vi "Parse Headers.vi"(8 "error in":errorcluster, 11 "Header-Body Data in":T1) -> (0 "error out":errorcluster, 2 "HTTP Status":T2, 3 "Header-Body Data out":T1)   [LabVIEW 2020, in "InfluxDB v2 Client.lvlib"]
doc: "Parses headers into the components:\n1) Code\n2) Status (Headers)"
uses:
  InfluxDB v2 Client.lvlib
  HTTP Status.ctl
  Header-Body Data.ctl
  <vilib>/regexp/Match Regular Expression.xnode
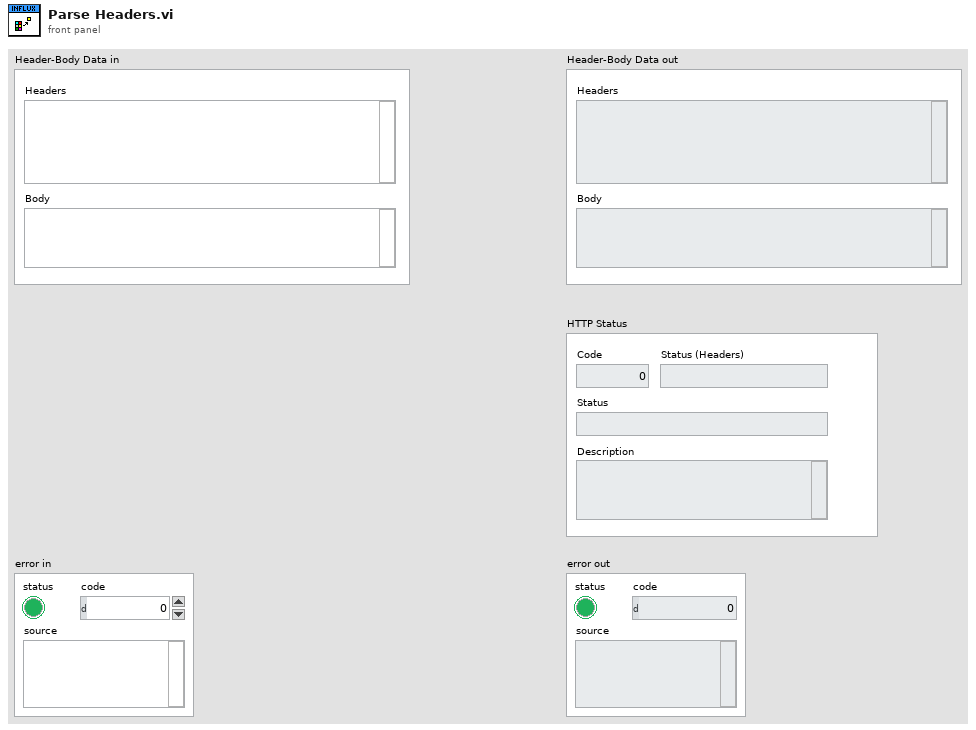
[diagram p1: front panel]
types:
  T1 = typedef "InfluxDB v2 Client.lvlib/Header-Body Data.ctl" = cluster{"Headers":string, "Body":string}
  T2 = typedef "InfluxDB v2 Client.lvlib/HTTP Status.ctl" = cluster{"Code":i32, "Status":string, "Description":string, "Status (Headers)":string}
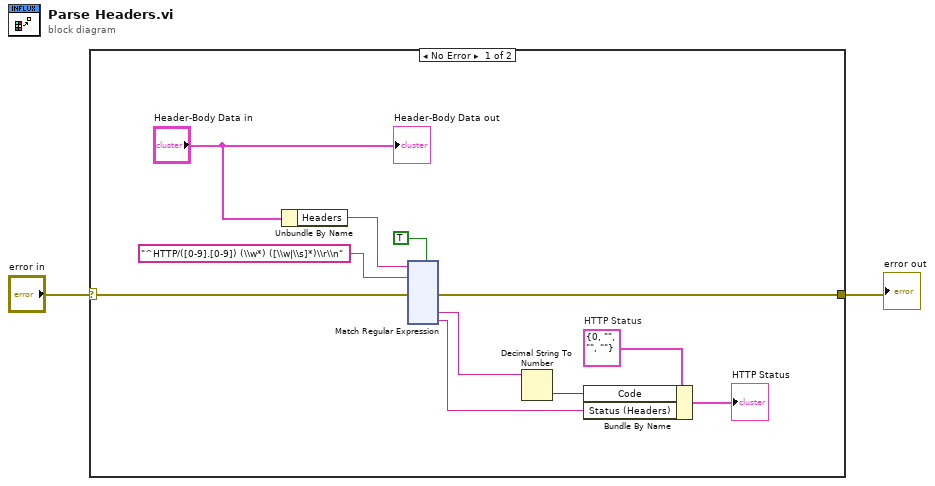
[diagram p0: block diagram]
diagram:
  n1 = case shown="No Error" "error in" {
    selector: "error in" -> [w10 w132]
    tunnel: [w4 w132] -> w1
    frame No Error {
      w8 = T2 {"Code"=0, "Status"="", "Description"="", "Status (Headers)"=""}  # HTTP Status
      n2 = Unbundle By Name("Header-Body Data in") -> ("Headers"=w11:string)
      n3 = xnode "Match Regular Expression"("input string"=w11, "regular expression"="^HTTP/([0-9].[0-9]) (\\w*) ([\\w|\\s]*)\\r\\n", "error in"=w10, "multiline? (F)"=TRUE) -> ("error out"=w4:errorcluster, "submatch 2"=w9:string, "submatch 3"=w5:string)  [unwired: 2 in, 5 out]
      n4 = Decimal String To Number(string=w9) -> (number=w6:i32)  [unwired: 2 in, 1 out]
      n5 = Bundle By Name(cluster=w8, "Code"=w6, "Status (Headers)"=w5) -> (→"HTTP Status":T2)
      "Header-Body Data out" <- "Header-Body Data in"
    }
    frame Error {
    }
  }
  "error out" <- w1
